vi "Init Actor.vi"() -> (3 "Base Actor out":refnum<class "Base Actor.lvclass">)   [LabVIEW 2025, in "jettl.lvlib" / "Base Actor.lvlib" / "Base Actor.lvclass"]
uses:
  Base Actor.lvclass
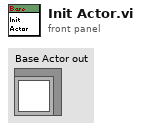
[diagram p1: front panel]
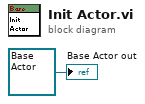
[diagram p0: block diagram]
diagram:
  "Base Actor out" <- refnum<class "Base Actor.lvclass"> refnum ("jettl Event Actor out")
